vi "VTI-RunRampT.vi"(1 "Rate (K/min)":dbl format="%#_13g", 2 "Final T (K)":dbl format="%#_13g") -> (0 "Current Setpoint":dbl format="%#_13g")   [LabVIEW 2019]
uses:
  Global/Global Variables/Data_Display_global.vi
  Instrument_Setup.vi
panel:
  out "K/s":dbl format="%#_13g"
  out "Sweep Time":dbl format="%#_13g"
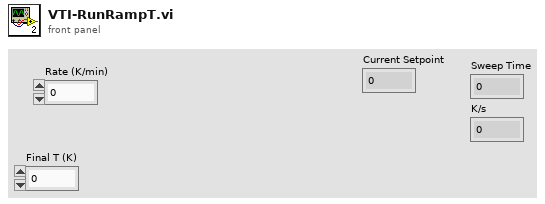
[diagram p1: front panel]
types:
  T1 = typedef "ITCVersion.ctl" = enum16{"ITC502", "ITC503", "ITC601"}
  T2 = cluster{"Version":T1, "ControlTITC":i8, "ControlTCh":i8, "SampleTITC":i8, "SampleTCh":i8, "Instrument address":cluster{"Com Port":i32, "ISOBUS Address":i32, "GPIB Address":i16, "Communication":enum16{"RS232", "ISOBUS", "GPIB", "Gateway"}}}
  T3 = cluster{"Com Port":i32, "ISOBUS Address":i32, "GPIB Address":i16, "Communication":enum16{"RS232", "ISOBUS", "GPIB", "Gateway"}}
  T4 = typedef "VTI-cluster.ctl" = cluster{"Temperatur (K)":dbl, "Setpoint (K)":dbl, "Rate (K/min)":dbl, "Heater (%)":dbl, "NV (%)":dbl, "Heater Manual":bool, "NV Manual":bool, "Go to Set":bool, "Pressure":dbl, "Heater SP":dbl, "Valid?":bool, "Set Heater SP":bool, "Set NV SP":bool, "Heater (%) Display":dbl, "NV (%) Display":dbl, "NV Setpoint":dbl, "Change Heater Status":bool, "Change NV Status":bool, "Sample 3":dbl, "Sample 2":dbl, "Sweep-State":bool, "Set Auto PID":bool, "Auto PID":bool, "Stopp":bool, "Setpoint-Sweep":dbl}
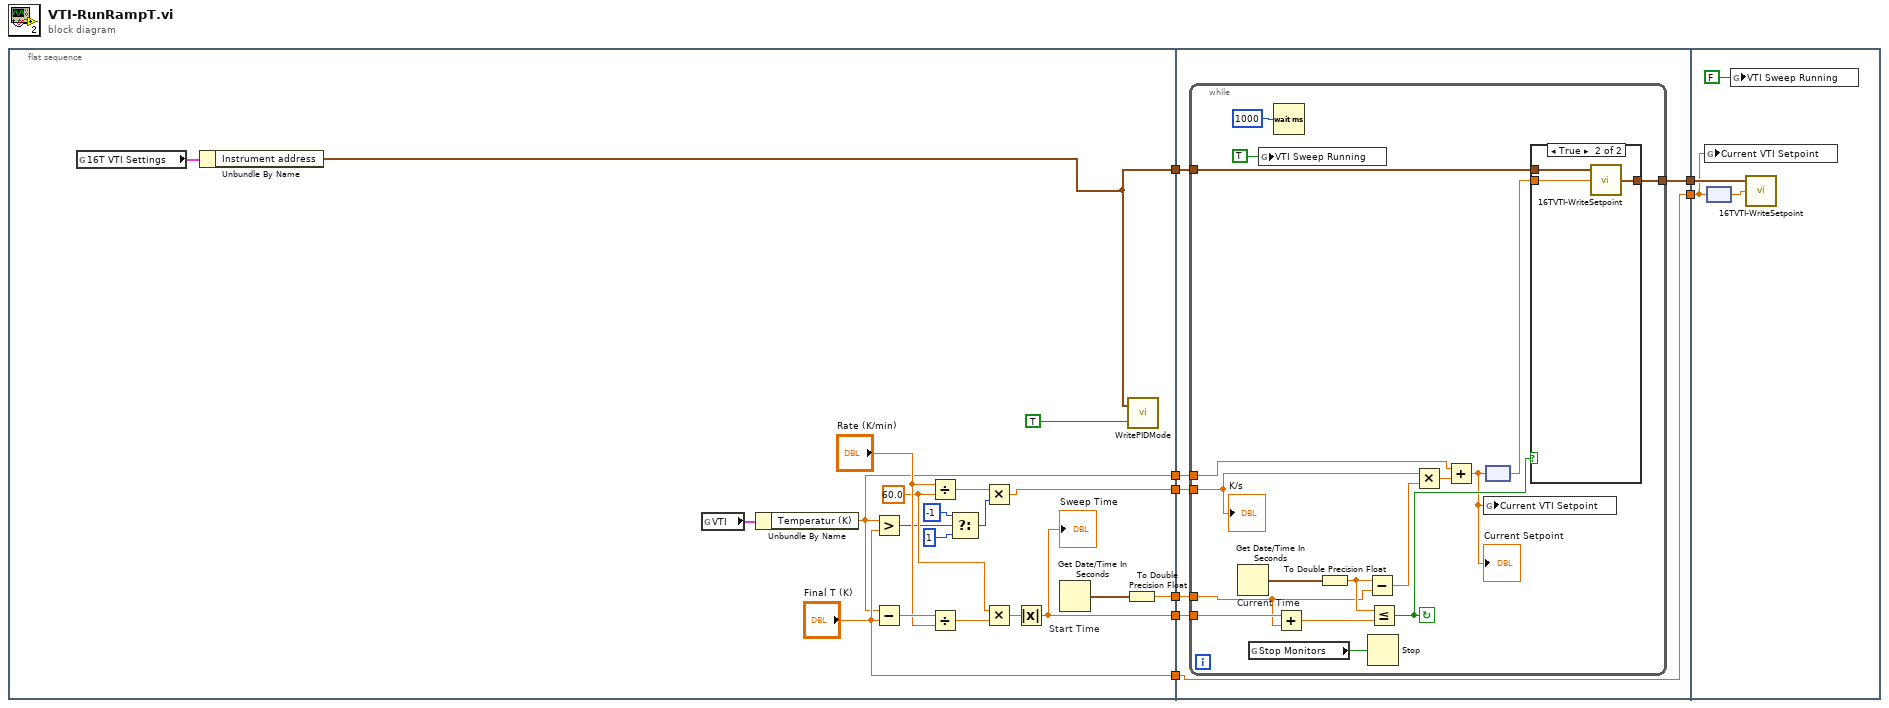
[diagram p0: block diagram]
diagram:
  n1 = flat-sequence {
    tunnel: [w12] -> w8
    tunnel: [w17] -> w7
    tunnel: [w25] -> w6
    tunnel: [w20] -> w5
    tunnel: ["Final T (K)"] -> w3
    tunnel: [w9] -> w2
    tunnel: w8 -> [w35]
    tunnel: w7 -> [w34]
    tunnel: w6 -> [w33]
    tunnel: w5 -> [w32]
    tunnel: [w31] -> w4
    tunnel: w3 -> [w31]
    tunnel: w2 -> [w30]
    tunnel: [w29] -> w1
    tunnel: w4 -> [w58]
    tunnel: w1 -> [w59]
    frame #0 {
      w22 = 60.0
      n2 = global read "Instrument_Setup.vi" "16T VTI Settings"() -> (w10:T2)
      n3 = Unbundle By Name(w10) -> ("Instrument address"=w9:T3)
      n4 = global read "Data_Display_global.vi" "VTI"() -> (w28:T4)
      n5 = Unbundle By Name(w28) -> ("Temperatur (K)"=w17:dbl)
      n6 = Greater?(x=w17, y="Final T (K)") -> (0:w16:bool)
      n7 = Subtract(x=w17, y="Final T (K)") -> (x-y=w27:dbl)
      n8 = Divide(x="Rate (K/min)", y=w22) -> (x/y=w13:dbl)
      n9 = Divide(x=w27, y="Rate (K/min)") -> (x/y=w23:dbl)
      n10 = Select(t=-1, s=w16, f=1) -> (s? t:f=w11:i32)
      n11 = Multiply(x=w13, y=w11) -> (x*y=w12:dbl)
      n12 = Multiply(x=w22, y=w23) -> (x*y=w21:dbl)
      n13 = Absolute Value(x=w21) -> (abs(x)=w20:dbl)
      "Sweep Time" <- w20
      n14 = Get Date/Time In Seconds "Start Time"() -> (seconds since 1Jan1904=w26:timestamp)
      n15 = To Double Precision Float(number=w26) -> (double precision float=w25:dbl)
      n16 = call "WritePIDMode.vi"("Auto PID"=TRUE, "Instrument address"=w9) -> ()  [unwired: 1 in, 1 out]
    }
    frame #1 {
      n17 = while {
        tunnel: w35 -> [w50]
        tunnel: w34 -> [w47]
        tunnel: w33 -> [w40]
        tunnel: w32 -> [w46]
        tunnel: w30 -> [w43]
        tunnel: [w42] -> w29
        stop <- w39 continue-if-true
        n18 = Get Date/Time In Seconds "Current Time"() -> (seconds since 1Jan1904=w52:timestamp)
        n19 = global read "Data_Display_global.vi" "Stop Monitors"() -> (w36:bool)
        n20 = global write "Data_Display_global.vi" "VTI Sweep Running"(TRUE) -> ()
        n21 = Wait (ms)(milliseconds to wait=1000) -> ()  [unwired: 1 out]
        n22 = Add(x=w46, y=w40) -> (x+y=w45:dbl)
        n23 = To Double Precision Float(number=w52) -> (double precision float=w41:dbl)
        n24 = Subtract(x=w41, y=w40) -> (x-y=w51:dbl)
        n25 = Stop(stop? (T)=w36) -> ()
        n26 = Less Or Equal?(x=w41, y=w45) -> (x <= y?=w39:bool)
        n27 = Multiply(x=w50, y=w51) -> (x*y=w49:dbl)
        n28 = Add(x=w47, y=w49) -> (x+y=w38:dbl)
        "Current Setpoint" <- w38
        n29 = global write "Data_Display_global.vi" "Current VTI Setpoint"(w38) -> ()
        n30 = node(w38) -> (w44:dbl[unit])
        n31 = case shown="True" w39 {
          tunnel: w44 -> [_ w56]
          tunnel: w43 -> [w53 w55]
          tunnel: [w53 w54] -> w42
          frame False {
          }
          frame True {
            n32 = call "16TVTI-WriteSetpoint.vi"("Set point"=w56, "Instrument address"=w55) -> ("Instrument address (out)"=w54:T3)  [unwired: 1 in]
          }
        }
        "K/s" <- w50
      }
    }
    frame #2 {
      n33 = global write "Data_Display_global.vi" "Current VTI Setpoint"(w58) -> ()
      n34 = node(w58) -> (w60:dbl[unit])
      n35 = global write "Data_Display_global.vi" "VTI Sweep Running"(FALSE) -> ()
      n36 = call "16TVTI-WriteSetpoint.vi"("Set point"=w60, "Instrument address"=w59) -> ()  [unwired: 1 in, 1 out]
    }
  }
